vi "Get Scan Engine Path.vi"(11 "ProjectItem in":refnum<vi>) -> (3 "Path":string)   [LabVIEW 2014, in "Scan Engine editor node.lvclass"]
uses:
  Scan Engine editor node.lvclass
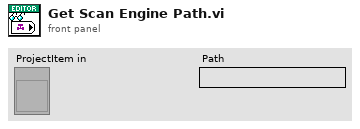
[diagram p1: front panel]
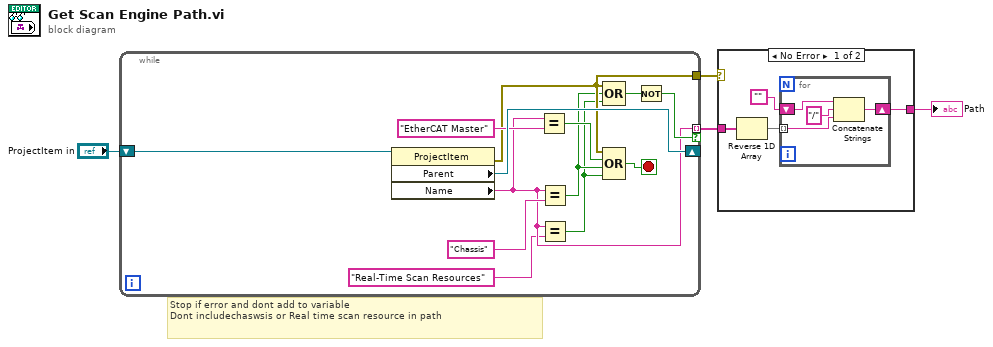
[diagram p0: block diagram]
diagram:
  # "Stop if error and dont add to variable\nDont includechaswsis or Real time scan resource in path"
  n1 = while {
    shift-right: [w16] -> _
    shift-left: "ProjectItem in" -> [w17]
    tunnel: [w7] -> w3 mode=indexing if=w9
    tunnel: [w11] -> w1
    stop <- w13 stop-if-true
    n2 = property class="ProjectItem"(reference=w17) -> (error out=w11:errorcluster, "Parent"=w16:refnum<vi>, "Name"=w7:string)  [unwired: 1 in, 1 out]
    n3 = Equal?(x=w7, y="EtherCAT Master") -> (x = y?=w14:bool)
    n4 = Equal?(x=w7, y="Chassis") -> (x = y?=w10:bool)
    n5 = Equal?(x=w7, y="Real-Time Scan Resources") -> (x = y?=w5:bool)
    n6 = Compound Arithmetic op=OR(w11, w10, w5) -> (w8:bool)
    n7 = Compound Arithmetic op=OR(w11, w14, w10, w5) -> (w13:bool)
    n8 = Not(x=w8) -> (.not. x?=w9:bool)
  }
  n9 = case shown="No Error" w1 {
    tunnel: w3 -> [w21 _]
    tunnel: [w19 _] -> w2
    frame No Error {
      n10 = Reverse 1D Array(array=w21) -> (reversed array=w20:string[])
      n11 = for {
        tunnel: w20 -> [w25] mode=indexing
        shift-right: [w23] -> w19
        shift-left: "" -> [w24]
        n12 = Concatenate Strings(w24, "/" ("string"), w25) -> (w23:string)
      }
    }
    frame Error {
    }
  }
  "Path" <- w2
